vi "阈值提醒.vi"(0 "添加的数组":bool[](array[boolean])) -> ()   [LabVIEW 2014]
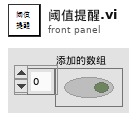
[diagram p1: front panel]
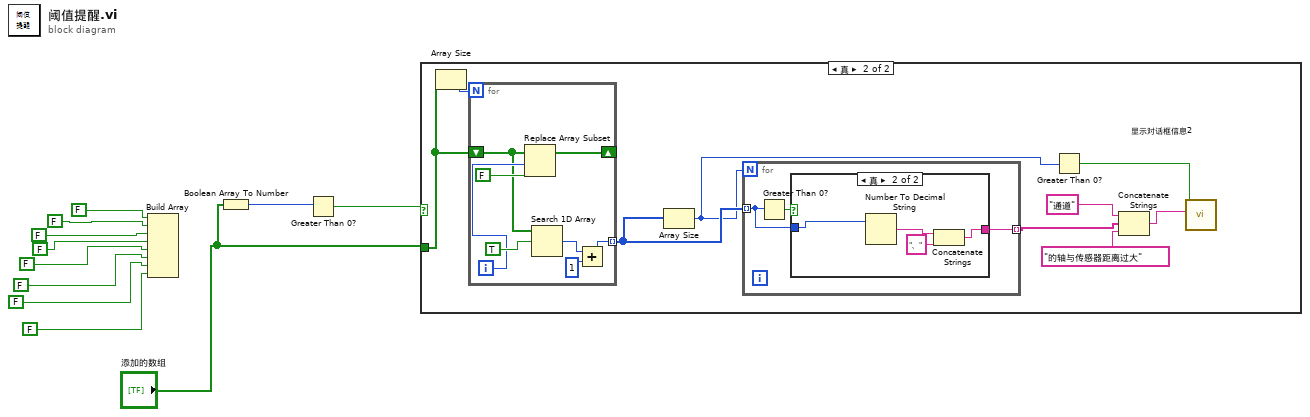
[diagram p0: block diagram]
diagram:
  n1 = Build Array(FALSE, FALSE, FALSE, FALSE, FALSE, FALSE, FALSE, FALSE) -> ()  [unwired: 1 out]
  n2 = Boolean Array To Number(Boolean array="添加的数组") -> (number=w3:u32)
  n3 = Greater Than 0?(x=w3) -> (x > 0?=w2:bool)
  n4 = case shown="真" w2 {
    tunnel: "添加的数组" -> [_ w20]
    frame False {
    }
    frame True {
      n5 = Array Size(array=w20) -> (size(s)=w19:i32)
      n6 = for {
        N: w19 -> [_]
        tunnel: [w28] -> w18 mode=indexing
        shift-right: [w32] -> _
        shift-left: w20 -> [w31]
        i -> [w33]
        n7 = Replace Array Subset(array=w31, new element=FALSE ("元素"), index=w33) -> (w32:bool[])
        n8 = Search 1D Array(1D array=w31, element=TRUE ("元素")) -> (index of element=w30:i32)  [unwired: 1 in]
        n9 = Add(x=w30, y=1) -> (x+y=w28:i32)
      }
      n10 = Array Size(array=w18) -> (size(s)=w12:i32)
      n11 = for {
        N: w12 -> [_]
        tunnel: w18 -> [w22] mode=indexing
        tunnel: [w21] -> w13 mode=indexing
        n12 = Greater Than 0?(x=w22) -> (x > 0?=w23:bool)
        n13 = case shown="真" w23 {
          tunnel: w22 -> [_ w25]
          tunnel: [_ w24] -> w21
          frame False {
          }
          frame True {
            n14 = Number To Decimal String(number=w25) -> (decimal integer string=w27:string)  [unwired: 1 in]
            n15 = Concatenate Strings(w27, "、") -> (w24:string)
          }
        }
      }
      n16 = Greater Than 0?(x=w12) -> (x > 0?=w14:bool)
      n17 = Concatenate Strings("通道", w13, "的轴与传感器距离过大") -> (w15:string)
      n18 = call "显示对话框信息2"("Enable"=w14, "Message"=w15) -> ()  [unwired: 8 in, 2 out]
    }
  }
